vi "String-Based Partial Loading.vi"() -> ()   [LabVIEW 2018]
doc: "Demonstrates compiling a logic-free mustache template with partial templates stored as strings."
uses:
  Toolkit/Data/Array/Array.lvclass
  D:/Users/cfield/Code/Field R&D Services/Labstache/src/Toolkit/Data/Datum/Datum.lvclass
  Toolkit/Low-Level/Loaders/String/String.lvclass
  D:/Users/cfield/Code/Field R&D Services/Labstache/src/Toolkit/Low-Level/Loaders/Loader/Loader.lvclass
  Toolkit/Data/Pair/Support/From String.vi
  Toolkit/Data/Array/Support/From Mapped Strings.vi
  Toolkit/Data/Pair/Support/From Datum.vi
  Toolkit/Support/Compile with Pair Array.vi
  Toolkit/Toolkit.lvlib
  Toolkit/Data/Pair/Pair.lvclass
panel:
  out "Output":string
  in  "Input":string="This is a simple mustache template.\n\n{{greeting}} {{person}}!\n\nAny kind of text, or string, can be created as a mustache template, but it is particularly useful for creating HTML files.\n\nHere is a list of different types of mustaches using HTML:\n\n{{>list}}"
  # "Overview: Demonstrates compiling a mustache template string with only variable tags\nInstructions:\n1. Run this VI"
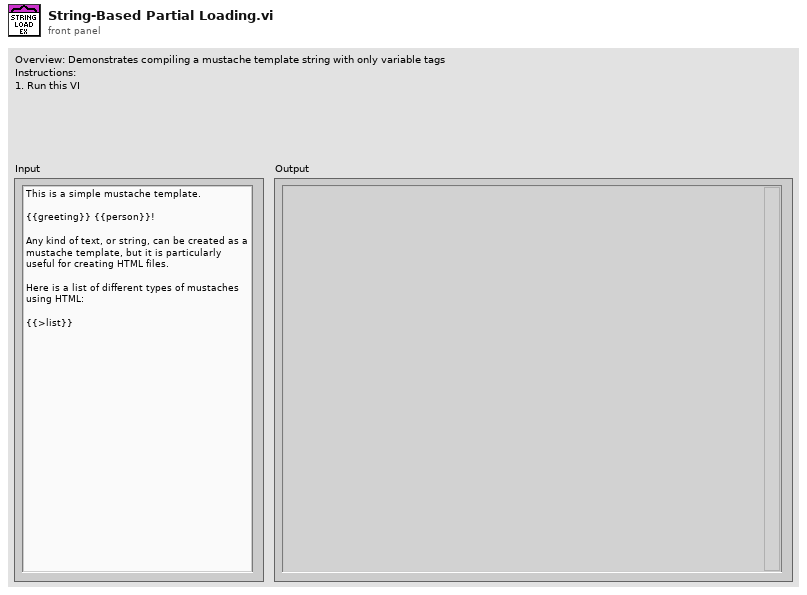
[diagram p1: front panel]
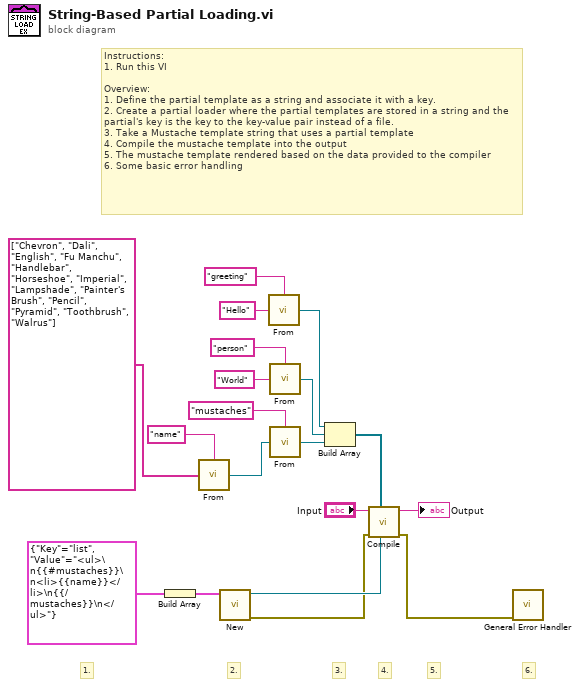
[diagram p0: block diagram]
diagram:
  # "6."
  # "Instructions:\n1. Run this VI\n\nOverview:\n1. Define the partial template as a string and associate it with a key.\n2. Create a partial loader where the partial templates are stored in a string and the partial's key is the key to the key-value pair instead of a file.\n3. Take a Mustache template string that uses a partial template\n4. Compile the mustache template into the output\n5. The mustache template rendered based on the data provided to the compiler\n6. Some basic error handling"
  # "5."
  # "4."
  # "3."
  # "2."
  # "1."
  n1 = Build Array(cluster{"Key":string, "Value":string} {"Key"="list", "Value"="<ul>\n{{#mustaches}}\n<li>{{name}}</li>\n{{/mustaches}}\n</ul>"} ("Key-Value Pair")) -> (w11:cluster{"Key":string, "Value":string}[])
  n2 = call-poly "From.vi"("Strings"=string[] ["Chevron", "Dali", "English", "Fu Manchu", "Handlebar", "Horseshoe", "Imperial", "Lampshade", "Painter's Brush", "Pencil", "Pyramid", "Toothbrush", "Walrus"], "Key"="name") -> ("Array"=w6:refnum<class "Array.lvclass">)
  n3 = call "New.vi"("Key-Value Pairs"=w11) -> ("Error Out"=w13:errorcluster, "String"=w16:refnum<class "String.lvclass">)  [unwired: 9 in]
  n4 = call-poly "From.vi"("Value"="Hello", "Key"="greeting") -> ("Pair"=w4:refnum<class "Pair.lvclass">)
  n5 = call-poly "From.vi"("Value"="World", "Key"="person") -> ("Pair"=w3:refnum<class "Pair.lvclass">)
  n6 = call-poly "From.vi"("Value"=w6, "Key"="mustaches") -> ("Pair"=w2:refnum<class "Pair.lvclass">)
  n7 = Build Array(w4, w3, w2) -> (w1:refnum<class "Pair.lvclass">[])
  n8 = call-poly "Compile.vi"("Loader"=w16, "Data"=w1, "Error In"=w13, "Input"="Input") -> ("Error Out"=w19:errorcluster, "Output"=→"Output":string)  [unwired: 6 in]
  n9 = call <vilib>:"General Error Handler.vi"("error in (no error)"=w19) -> ()  [unwired: 10 in, 5 out]
